vi "fill between last new.vi"(6 "value":dbl, 9 "array in":dbl[](array[numeric]), 10 "New":i32, 11 "Last":i32) -> (3 "array out":dbl[](array[numeric]))   [LabVIEW 2024]
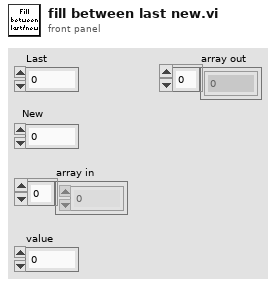
[diagram p1: front panel]
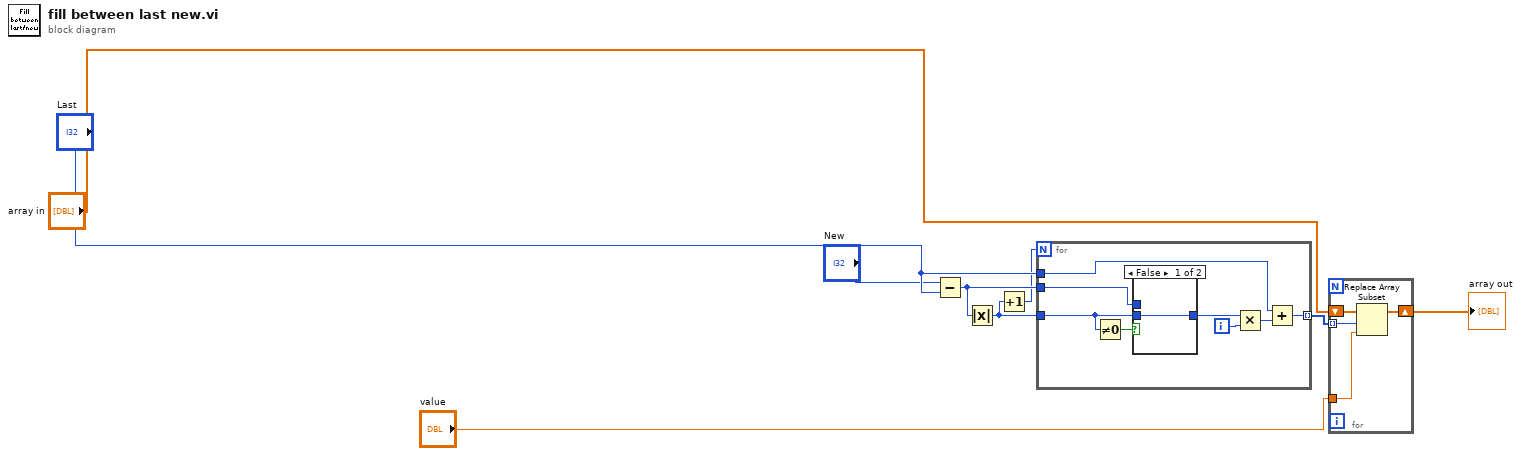
[diagram p0: block diagram]
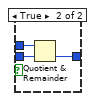
[diagram p2: hidden frame]
diagram:
  n1 = Subtract(x="New", y="Last") -> (x-y=w7:i32)
  n2 = Absolute Value(x=w7) -> (abs(x)=w8:i32)
  n3 = Increment(x=w8) -> (x+1=w5:i32)
  n4 = for {
    N: w5 -> [_]
    tunnel: "Last" -> [w17]
    tunnel: w7 -> [w14]
    tunnel: w8 -> [w11]
    tunnel: [w12] -> w9 mode=indexing
    i -> [w16]
    n5 = Not Equal To 0?(x=w11) -> (x != 0?=w10:bool)
    n6 = case shown="False" w10 {
      tunnel: w14 -> [_ w21]
      tunnel: w11 -> [w18 w20]
      tunnel: [w18 w19] -> w13
      frame False {
      }
      frame True {
        n7 = Quotient & Remainder(x=w21, y=w20) -> (floor(x/y)=w19:i32)  [unwired: 1 out]
      }
    }
    n8 = Multiply(x=w13, y=w16) -> (x*y=w15:i32)
    n9 = Add(x=w17, y=w15) -> (x+y=w12:i32)
  }
  n10 = for {
    tunnel: "value" -> [w23]
    tunnel: w9 -> [w22] mode=indexing
    shift-right: [w24] -> w2
    shift-left: "array in" -> [w25]
    n11 = Replace Array Subset(array=w25, new element=w23, index=w22) -> (w24:dbl[])
  }
  "array out" <- w2
